vi "Read File+ [I16]FixEOL.vi"(6 "2D number of columns/1D count":i32, 7 "2D number of rows":i32, 8 "error in (no error)":errorcluster, 9 "pos offset (bytes:0)":i32, 10 "pos mode (rel. to current:2)":enum16{"start", "end", "current"}(ring)=enum."current", 11 "refnum":refnum<file>) -> (0 "error out":errorcluster, 1 "mark after read (bytes)":i32, 2 "1D data":i16[](array[numeric]), 4 "EOF?":bool, 5 "dup refnum":refnum<file>)   [LabVIEW 2020]
doc: "Reads a 2D or 1D array of signed word integers (I16) from a byte stream file at the specified location; the default location is at the current mark. The VI does incoming and internal error checking and does not read if an incoming error occurs.\n\nrefnum is the reference number of the open file.\n\npos mode specifies where the read begins relative to pos offset:\n\n 0: at the beginning of the file plus pos offset.\n\n 1: at the end of the file plus pos offset. \n\n 2: at the current file mark plus pos offset. This is the default value.\n\npos offset specifies in bytes how far from the location specified by pos mode that the operation begins. The default value is 0. Byte units rather than integer (2 byte) units for flexibility, for example, so that a file can contain a text header written with Write File+ (string) followed by arrays of number written with Write File+ [I16].\n\n2D number of rows is the number of rows to create if the data is to be returned in the 2D array output. If the value is 0 (default), the data is returned in the 1D array.\n\n2D number of columns/1D count is the number of columns to create if the data is to be returned in the 2D array output, provided that 2D number of rows is >0; otherwise, this is the number of signed word integers to read and return in the 1D array output.\n\nerror in is a cluster of three elements (error?, code, and source) that describe the upstream error state, that is, the existance of any error preceeding the execution of the VI. The VI executes normally only if no incoming error exists; otherwise it merely passes the error in value to error out. error? is TRUE if an error occurred; the default value is FALSE. code is the error code; the default value is 0. source is in most cases the name of the VI or function that produced the error; the default value is an empty string.\n\ndup refnum is a flow-though parameter with the same value as refnum.\n\n2D array contains the signed word integers read from the file if 2D number of rows is greater than 0; otherwise, this output is empty.\n\n1D array contains the signed word integers read from the file if 2D number of rows equal 0; otherwise, this output is empty.\n\nmark after read is the location of the file mark after the read; it points to the byte in the file following the last byte read.\n\nEOF? is TRUE if you attempt to read past the end of file.\n\nerror out is a cluster of three elements (error?, code, and source) that describe the error state following the execution of the VI. If an incoming error does not exist, the VI executes normally and error out describes the VI's error state; if an incoming error exists, error out equals error in."
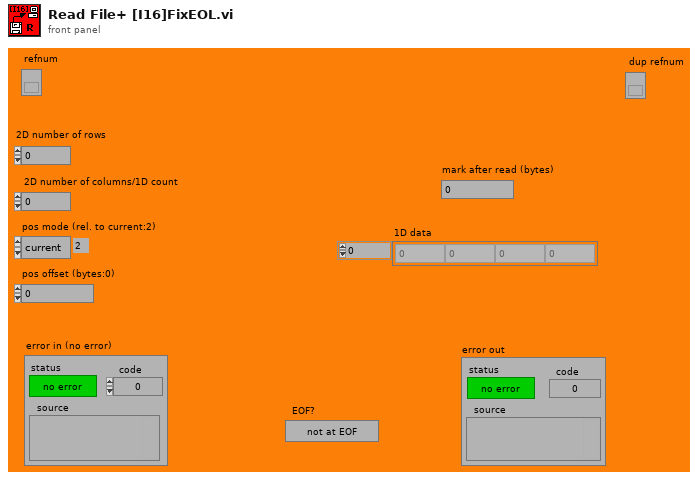
[diagram p1: front panel]
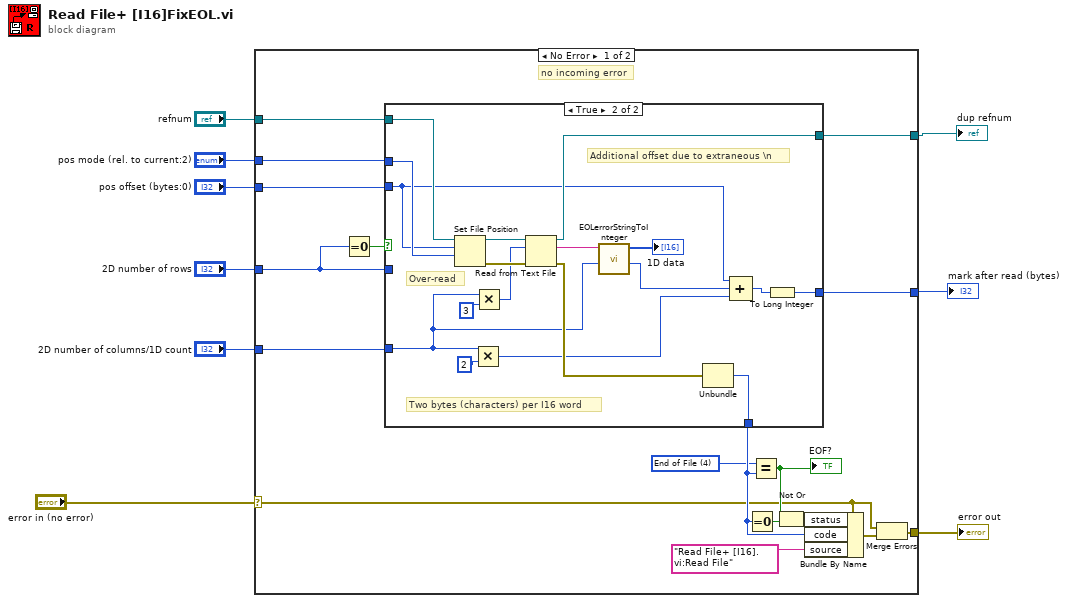
[diagram p0: block diagram]
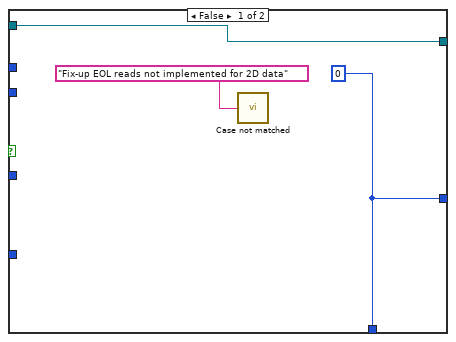
[diagram p2: hidden frame]
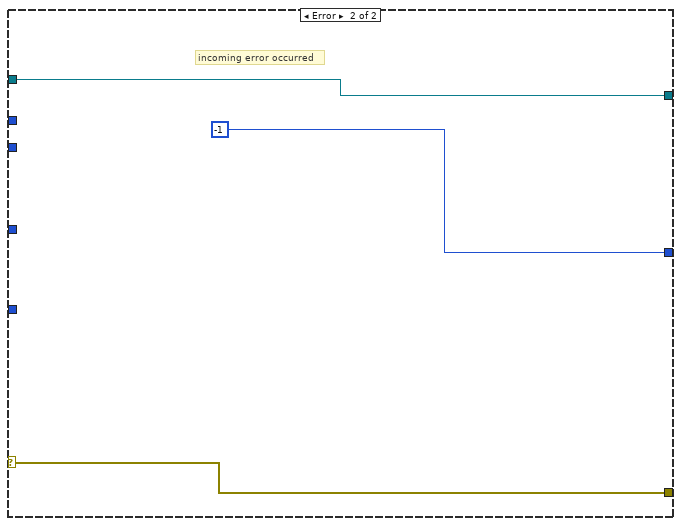
[diagram p3: hidden frame]
diagram:
  n1 = case shown="No Error" "error in (no error)" {
    selector: "error in (no error)" -> [w10 w48]
    tunnel: [w16 w48] -> w9
    tunnel: [w23 -1] -> w8
    tunnel: [w25 w49] -> w7
    tunnel: "refnum" -> [w24 w49]
    tunnel: "2D number of columns/1D count" -> [w14 _]
    tunnel: "2D number of rows" -> [w13 _]
    tunnel: "pos offset (bytes:0)" -> [w12 _]
    tunnel: "pos mode (rel. to current:2)" -> [w11 _]
    frame No Error {
      w18 = 4 items=["No Error", "Manager Argument Error", "Memory Full", "Out of Zone", "End of File", "File Already Open", "Generic File IO Error", "File Not Found", "File Permission Error", "Disk Full", "Duplicate Path", "Too Many Files Open", "Not Enabled", "Resource File Not Found", "Cannot Add Resource", "Resource Not Found", "Image Not Found", "Image Memory Error", "Pen Does Not Exist", "Config Bad Type", "Config Token Not Found", "Config Parse Error", "Config Memory Error", "Bad External Code Format", "Bad External Code Offset", "External Code Not Present", "Null Window", "Destroy Window Mixup", "Null Menu", "Print Aborted", "Bad Print Record", "Print Driver Error", "Windows Error During Print", "Memory Error During Print", "Print Dialog Error", "Generic Print Error", "Invalid Device Refnum", "Device Not Found", "Device Parameter Error", "Device Unit Error", "Can't Open Device", "Device Call Aborted", "Generic Error", "Cancelled By User", "Object ID Too Low", "Object ID Too High", "Object Not In Heap", "Unknown Heap", "Bad DefProc ID", "DefProc Not In Table", "Message Out Of Range", "Null Method", "Unknown Message", "Manager Call Not Supported"]
      # "no incoming error"
      n2 = Equal To 0?(x=w13) -> (x = 0?=w26:bool)
      n3 = case shown="True" w26 {
        tunnel: [w28 w41] -> w20
        tunnel: [w28 w47] -> w23
        tunnel: w14 -> [_ w31]
        tunnel: w13 -> [_ _]
        tunnel: [w29 w45] -> w25
        tunnel: w24 -> [w29 w37]
        tunnel: w11 -> [_ w42]
        tunnel: w12 -> [_ w30]
        frame False {
          w28 = 0
          n4 = call "Case not matched.vi"("Case Name not Matched"="Fix-up EOL reads not implemented for 2D data") -> ()
        }
        frame True {
          # "Two bytes (characters) per I16 word"
          # "Over-read"
          # "Additional offset due to extraneous \\n"
          n5 = Set File Position(offset (in bytes) (0)=w30, refnum=w37, from (0:start)=w42) -> (refnum out=w46:refnum<file>, error out=w44:errorcluster)  [unwired: 1 in]
          n6 = Multiply(x=w31, y=2) -> (x*y=w34:i32)
          n7 = Multiply(x=w31, y=3) -> (x*y=w40:i32)
          n8 = Read from Text File(file (use dialog)=w46, count=w40, error in=w44) -> (refnum out=w45:refnum<file>, text=w38:string, error out=w43:errorcluster)  [unwired: 1 in, 1 out]
          n9 = call "EOLerrorStringToInteger.vi"("targetLength"=w31, "binaryString"=w38) -> ("\\nRemoved"=w32:i32, "trimmedSelectiveReplaceData"=→"1D data":i16[])  [unwired: 8 in]
          n10 = Unbundle(w43) -> ("code"=w41:i32)  [unwired: 2 out]
          n11 = Compound Arithmetic op=ADD(w30, w32, w34) -> (w33:i32)
          n12 = To Long Integer(number=w33) -> (32bit integer=w47:i32)
        }
      }
      n13 = Equal To 0?(x=w20) -> (x = 0?=w22:bool)
      n14 = Equal?(x=w18, y=w20) -> (x = y?=w21:bool)
      "EOF?" <- w21
      n15 = Not Or(1:w22, 2:w21) -> (0:w17:bool)
      n16 = Bundle By Name(cluster=w10, "status"=w17, "code"=w20, "source"="Read File+ [I16].vi:Read File") -> (w15:errorcluster)
      n17 = Merge Errors(w10, w15) -> (w16:errorcluster)
    }
    frame Error {
      # "incoming error occurred"
    }
  }
  "error out" <- w9
  "mark after read (bytes)" <- w8
  "dup refnum" <- w7
